vi "Write.ProcessData.vi"(8 "error in (no error)":errorcluster, 10 "Values":dbl[](array[numeric]), 11 "Write in":refnum<class "Write.lvclass">) -> (0 "error out":errorcluster, 3 "Write out":refnum<class "Write.lvclass">)   [LabVIEW 2015, in "Data Access API.lvlib" / "Write.lvclass"]
uses:
  Write.lvclass
  Write.lvclass/Write.ctl
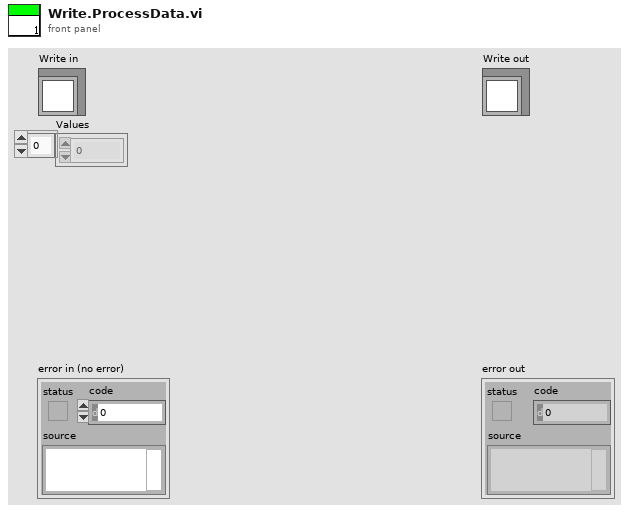
[diagram p1: front panel]
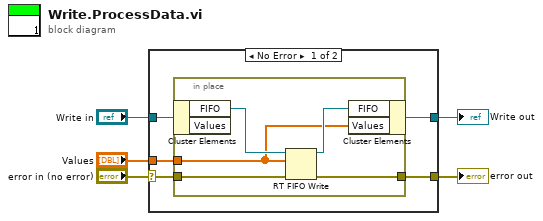
[diagram p0: block diagram]
diagram:
  n1 = case shown="No Error" "error in (no error)" {
    selector: "error in (no error)" -> [w7 w17]
    tunnel: [w6 w17] -> w4
    tunnel: [w9 w16] -> w2
    tunnel: "Write in" -> [w10 w16]
    tunnel: "Values" -> [w8 _]
    frame No Error {
      n2 = in-place {
        in-place-border: w8 -> [w13]
        in-place-border: w7 -> [w12]
        in-place-border: [w11] -> w6
        n3 = in-place-cluster #1(w10) -> ("FIFO"=w15:refnum<k33>)  [unwired: 1 out]
        n4 = RT FIFO Write(0:w15, 1:w13, 3:w12) -> (8:w14:refnum<k33>, 11:w11:errorcluster)  [unwired: 2 in, 2 out]
        n5 = in-place-cluster #1("FIFO"=w14, "Values"=w13) -> (w9:refnum<class "Write.lvclass">)
      }
    }
    frame Error {
    }
  }
  "error out" <- w4
  "Write out" <- w2
